vi "Get Number by Index.vi"(1 "Test Table":string[](array[string]), 2 "Index":i32=2) -> (0 "Dwell Time":dbl)   [LabVIEW 2018]
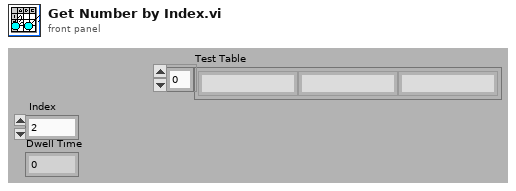
[diagram p1: front panel]
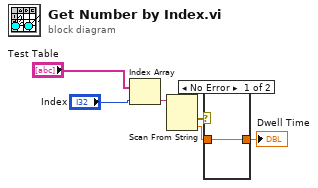
[diagram p0: block diagram]
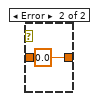
[diagram p2: hidden frame]
diagram:
  n1 = Index Array(array="Test Table", index="Index") -> (element=w5:string)
  n2 = Scan From String(input string=w5) -> (error out=w3:errorcluster, output 1=w6:dbl)  [unwired: 4 in, 2 out]
  n3 = case shown="No Error" w3 {
    tunnel: w6 -> [w7 _]
    tunnel: [w7 0.0] -> w2
    frame No Error {
    }
    frame Error {
    }
  }
  "Dwell Time" <- w2
